vi "teste.vi"() -> ()   [LabVIEW 2016]
panel:
  out "Gauge":dbl(knob) scale=0.0..10.0
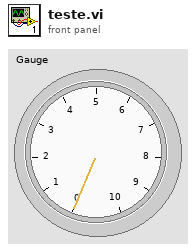
[diagram p1: front panel]
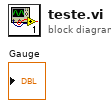
[diagram p0: block diagram]
diagram:
